vi "Write session data.vi"(8 "error in (no error)":errorcluster, 10 "session data":refnum<data-value>, 11 "LIA Host Interface FPGA in":refnum<class "LIA Host Interface FPGA.lvclass">) -> (0 "error out":errorcluster, 3 "LIA Host Interface FPGA out":refnum<class "LIA Host Interface FPGA.lvclass">)   [LabVIEW 2018, in "LIA Host Interface FPGA.lvclass"]
uses:
  LIA Host Interface FPGA.lvclass
  Session Data.ctl
  LIA Host Interface FPGA.lvclass/LIA Host Interface FPGA.ctl
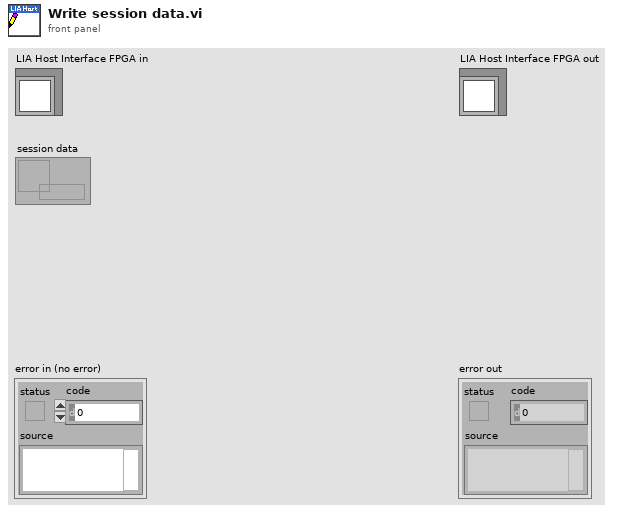
[diagram p1: front panel]
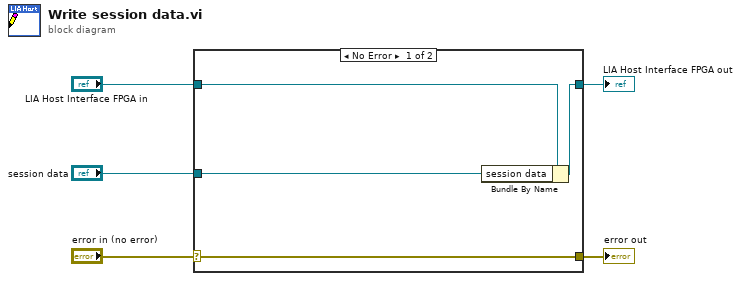
[diagram p0: block diagram]
diagram:
  n1 = case shown="No Error" "error in (no error)" {
    selector: "error in (no error)" -> [w9 w10]
    tunnel: [w9 w10] -> w4
    tunnel: [w7 w11] -> w2
    tunnel: "LIA Host Interface FPGA in" -> [w8 w11]
    tunnel: "session data" -> [w6 _]
    frame No Error {
      n2 = Bundle By Name(cluster=w8, "session data"=w6) -> (w7:refnum<class "LIA Host Interface FPGA.lvclass">)
    }
    frame Error {
    }
  }
  "error out" <- w4
  "LIA Host Interface FPGA out" <- w2
